vi "Recieve.vi"(7 "Message Priority":T1=enum."Normal", 8 "error in (no error)":errorcluster, 9 "Message":refnum<class "Message.lvclass">, 10 "Actor in":refnum<class "Actor.lvclass">, 11 "Sequencer Core in":refnum<class "Sequencer Core.lvclass">) -> (0 "error out":errorcluster, 2 "Actor out":refnum<class "Actor.lvclass">, 3 "Sequencer Core out":refnum<class "Sequencer Core.lvclass">)   [LabVIEW 2020, in "Sequencer.lvlib" / "Sequencer Core.lvclass"]
doc: "Non dynamic dispatch wrapper for 'Recieve Message'."
uses:
  Sequencer Core.lvclass
  PPL/HDH.Actor Framework.Core.Actor.lvlibp/1abvi3w/vi.lib/ActorFramework/Message Enqueuer/Message Priority.ctl
  PPL/HDH.Actor Framework.Core.Actor.lvlibp/1abvi3w/vi.lib/ActorFramework/Message/Message.lvclass
  PPL/HDH.Actor Framework.Core.Actor.lvlibp/1abvi3w/vi.lib/ActorFramework/Actor/Actor.lvclass
  PPL/HDH.Actor Framework.Core.Actor.lvlibp/1abvi3w/vi.lib/ActorFramework/Message Enqueuer/Message Enqueuer.lvclass
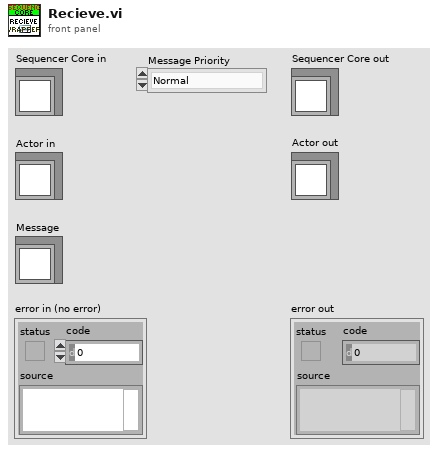
[diagram p1: front panel]
types:
  T1 = typedef "HDH.Actor Framework.Core.Actor.lvlibp/Message Enqueuer.lvclass/Message Priority.ctl" = enum16{"Low", "Normal", "High"}
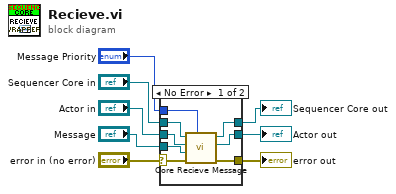
[diagram p0: block diagram]
diagram:
  n1 = case shown="No Error" "error in (no error)" {
    selector: "error in (no error)" -> [w10 w19]
    tunnel: [w9 w19] -> w7
    tunnel: [w15 w18] -> w5
    tunnel: "Sequencer Core in" -> [w16 w18]
    tunnel: "Actor in" -> [w12 w17]
    tunnel: "Message" -> [w13 _]
    tunnel: [w11 w17] -> w2
    tunnel: "Message Priority" -> [w14 _]
    frame No Error {
      n2 = call-dynamic "Core Recieve Message.vi"("Message Priority"=w14, "error in (no error)"=w10, "Message"=w13, "Actor in"=w12, "Sequencer Core in"=w16) -> ("error out"=w9:errorcluster, "Actor out"=w11:refnum<class "Actor.lvclass">, "Sequencer Core out"=w15:refnum<class "Sequencer Core.lvclass">)  [unwired: 4 in]
    }
    frame Error {
    }
  }
  "error out" <- w7
  "Sequencer Core out" <- w5
  "Actor out" <- w2
